vi "ble_cmd_gap_set_scan_parameters.vi"(6 "Scanning Technique":T1=1 items=["Pasive", "Active"], 8 "error in (no error)":errorcluster, 9 "Scan Window (125ms)":u16=125, 10 "Scan Interval (125ms)":u16=125, 11 "COM Bluegiga in":refnum<visa-resource-name>) -> (0 "error out":errorcluster, 3 "COM Bluegiga out":refnum<visa-resource-name>)   [LabVIEW 2013]
uses:
  type_def/scanning_technique.ctl
  type_def/message_class.ctl
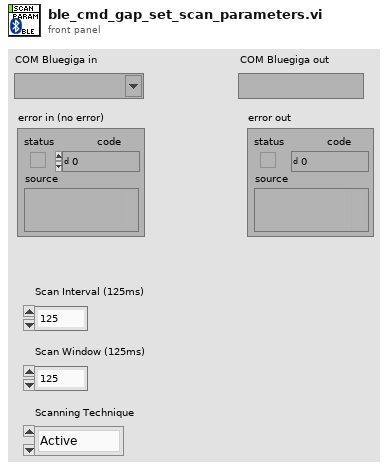
[diagram p1: front panel]
types:
  T1 = typedef "scanning_technique.ctl" = u8
  T2 = typedef "message_class.ctl" = u8
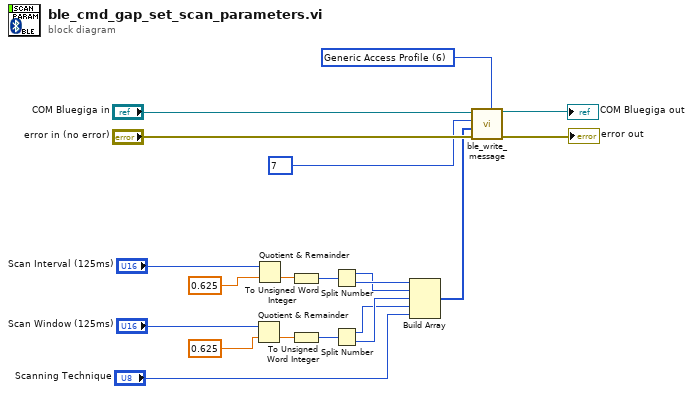
[diagram p0: block diagram]
diagram:
  w3 = T2 6 items=["System", "Persistent Store", "Attribute database", "Connection", "Attribute client", "Security Manager", "Generic Access Profile", "Hardware"] ("Command Class (System)")
  n1 = Quotient & Remainder(x="Scan Window (125ms)", y=0.625) -> (floor(x/y)=w12:dbl)  [unwired: 1 out]
  n2 = Quotient & Remainder(x="Scan Interval (125ms)", y=0.625) -> (floor(x/y)=w13:dbl)  [unwired: 1 out]
  n3 = To Unsigned Word Integer(number=w13) -> (unsigned 16bit integer=w11:u16)
  n4 = To Unsigned Word Integer(number=w12) -> (unsigned 16bit integer=w8:u16)
  n5 = Split Number(x=w11) -> (hi(x)=w9:u8, lo(x)=w10:u8)
  n6 = Split Number(x=w8) -> (hi(x)=w6:u8, lo(x)=w7:u8)
  n7 = Build Array(w10, w9, w7, w6, "Scanning Technique") -> (w4:T1[])
  n8 = call "ble_write_message.vi"("Command Class (System)"=w3, "error in (no error)"="error in (no error)", "Payload(Empty)"=w4, "Message ID (0x00)"=u8 7, "COM Bluegiga in"="COM Bluegiga in") -> ("error out"=→"error out":errorcluster, "COM Bluegiga out"=→"COM Bluegiga out":refnum<visa-resource-name>)  [unwired: 4 in, 1 out]
